vi "z query parameters.vi"(8 "error in (no error)":errorcluster, 10 "parameters":cluster{}, 11 "this_":cluster{}) -> (0 "error out":errorcluster, 2 "parameters out":cluster{})   [LabVIEW 2021, in "zenohc.lvlib"]
doc: "void z_query_parameters(const struct z_loaned_query_t *this_,\n struct z_view_string_t *parameters);"
uses:
  zenohc.lvlib
  zenohc.dll
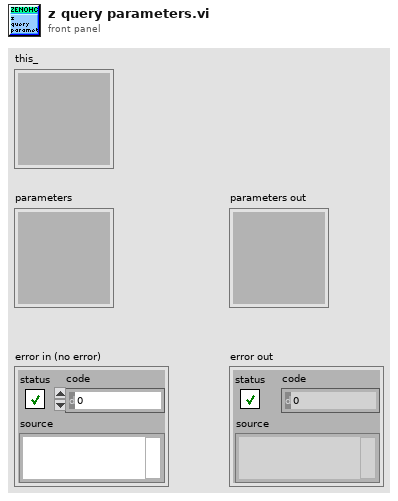
[diagram p1: front panel]
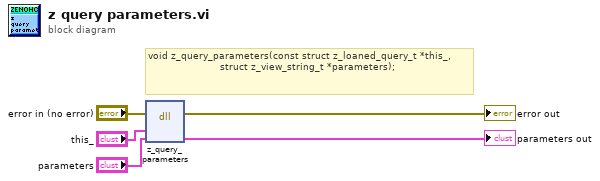
[diagram p0: block diagram]
diagram:
  # "void z_query_parameters(const struct z_loaned_query_t *this_,\n                        struct z_view_string_t *parameters);"
  n1 = dll-call lib="D:/dev/zenoh_labview/zenohc/zenohc.*" fn="z_query_parameters"(error in="error in (no error)", "this_"="this_", "parameters"="parameters") -> (error out=→"error out":errorcluster, "parameters"=→"parameters out":cluster{})  [unwired: 4 in, 1 out]
